vi "STS_Connect.vi"(8 "error in":errorcluster, 11 "Address Cluster out输入":T1 {"tsl_communcation_method" items=["GPIB", "C232C", "TCPIP", "USB"]; "MPM_communcation_method" items=["GPIB", "C232C", "TCPIP", "USB"]}) -> (0 "error out":errorcluster, 3 "Address Cluster out":T1 {"tsl_communcation_method" items=["GPIB", "C232C", "TCPIP", "USB"]; "MPM_communcation_method" items=["GPIB", "C232C", "TCPIP", "USB"]})   [LabVIEW 2017]
uses:
  CTL/Address Cluster.ctl
  D:/test/ILSTS/LV_IL_Sample/DLL/InstrumentDLL.dll
  DLL/InstrumentDLL.dll
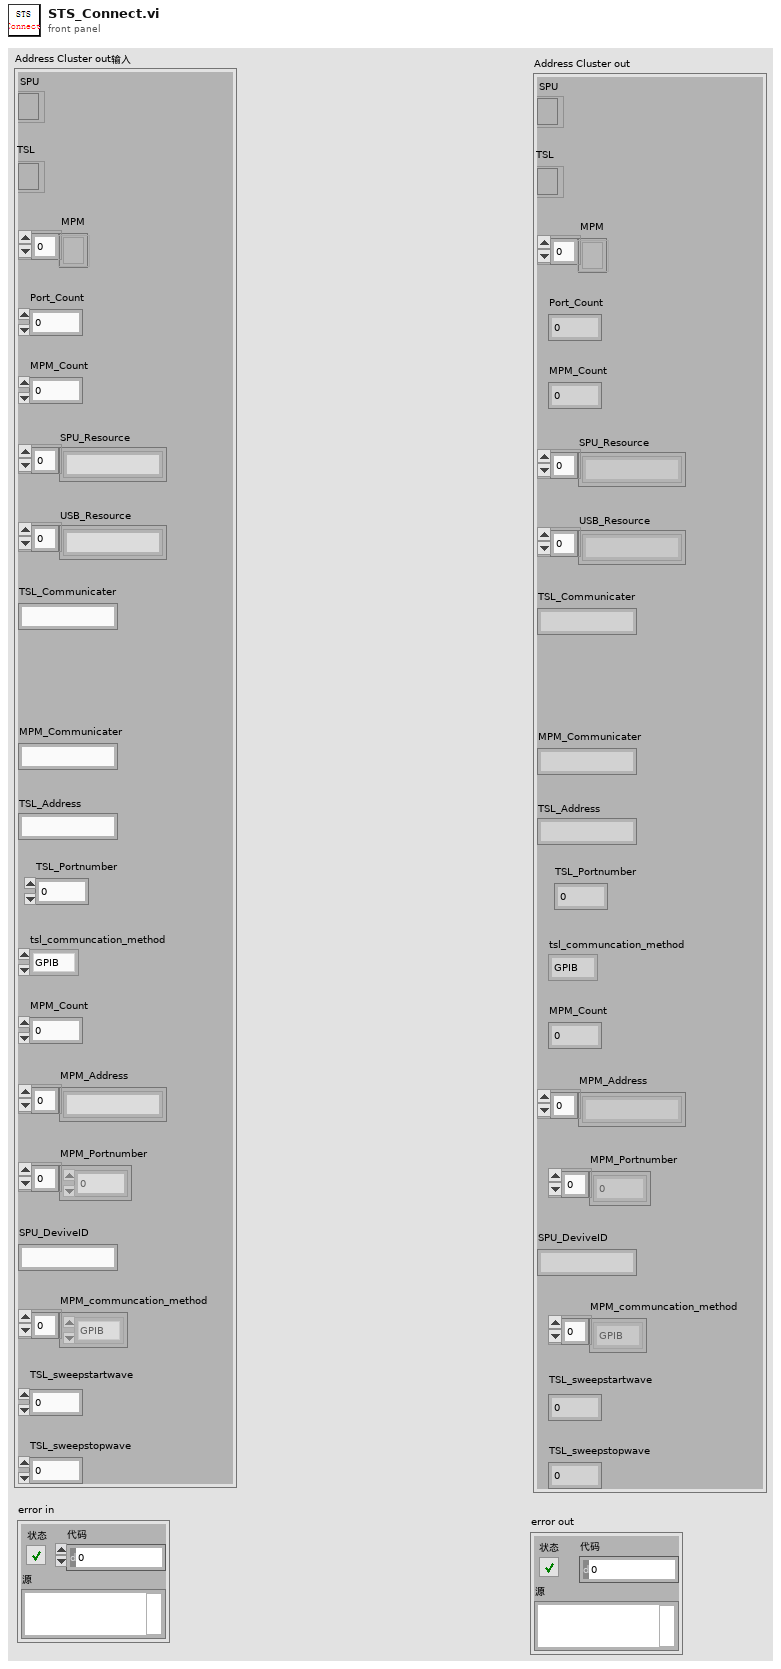
[diagram p1: front panel]
types:
  T1 = typedef "Address Cluster.ctl" = cluster{"SPU":refnum<k24>, "MPM":refnum<k24>[], "Port_Count":dbl, "MPM_Count":dbl, "SPU_Resource":string[], "USB_Resource":string[], "MPM_Communicater":string, "MPM_Count":dbl, "MPM_Address":string[], "MPM_Portnumber":dbl[], "SPU_DeviveID":string, "MPM_communcation_method":i32[], "TSL_sweepstartwave":dbl, "TSL_sweepstopwave":dbl, "TSL_Address":string, "TSL_Communicater":string, "TSL":refnum<k24>, "tsl_communcation_method":i32, "TSL_Portnumber":dbl}
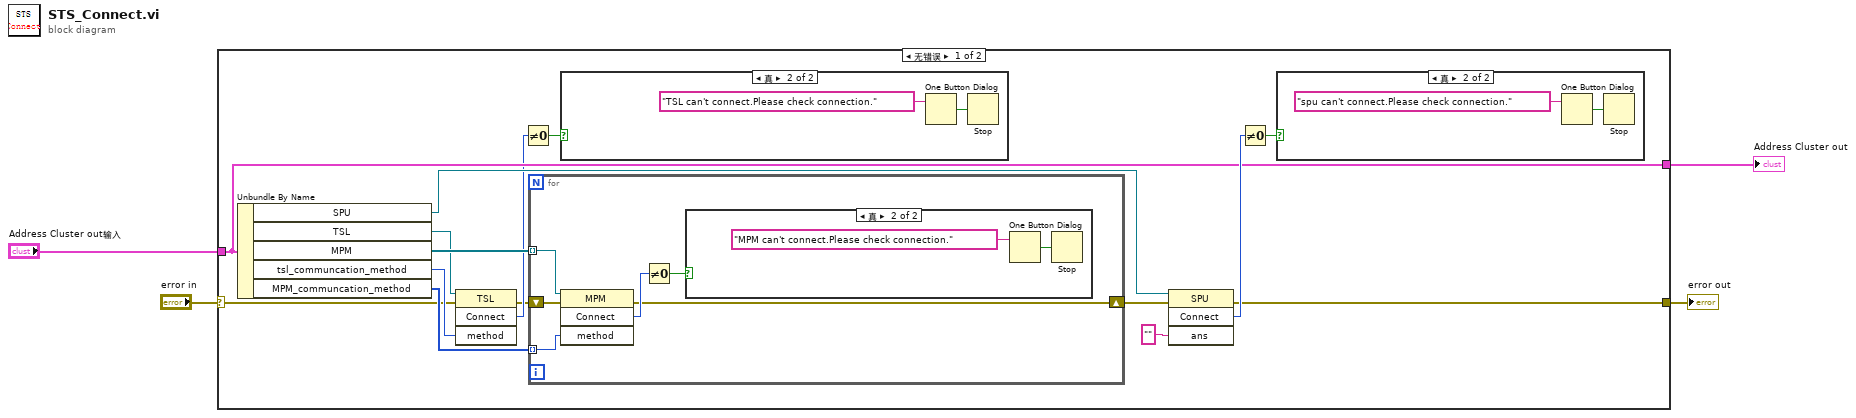
[diagram p0: block diagram]
diagram:
  n1 = case shown="无错误" "error in" {
    selector: "error in" -> [w11 w33]
    tunnel: "Address Cluster out输入" -> [w10 w32]
    tunnel: [w5 w33] -> w2
    tunnel: [w10 w32] -> w1
    frame No Error {
      n2 = Unbundle By Name(w10) -> ("SPU"=w17:refnum<k24>, "TSL"=w13:refnum<k24>, "MPM"=w15:refnum<k24>[], "tsl_communcation_method"=w14:i32, "MPM_communcation_method"=w16:i32[])
      n3 = invoke on="调用节点" class="TSL" method="Connect"(reference=w13, error in=w11, "method"=w14) -> (error out=w7:errorcluster, "Connect"=w9:i32)  [unwired: 1 in, 2 out]
      n4 = Not Equal To 0?(x=w9) -> (x != 0?=w8:bool)
      n5 = for {
        tunnel: w15 -> [w29] mode=indexing
        tunnel: w16 -> [w28] mode=indexing
        shift-right: [w25] -> w6
        shift-left: w7 -> [w24]
        n6 = invoke on="调用节点" class="MPM" method="Connect"(reference=w29, error in=w24, "method"=w28) -> (error out=w25:errorcluster, "Connect"=w26:i32)  [unwired: 1 in, 2 out]
        n7 = Not Equal To 0?(x=w26) -> (x != 0?=w27:bool)
        n8 = case shown="真" w27 {
          frame False {
          }
          frame True {
            n9 = One Button Dialog(message="MPM can't connect.Please check connection." ("消息")) -> (true=w30:bool)  [unwired: 1 in]
            n10 = Stop(stop? (T)=w30) -> ()
          }
        }
      }
      n11 = case shown="真" w8 {
        frame False {
        }
        frame True {
          n12 = One Button Dialog(message="TSL can't connect.Please check connection." ("消息")) -> (true=w20:bool)  [unwired: 1 in]
          n13 = Stop(stop? (T)=w20) -> ()
        }
      }
      n14 = invoke class="SPU" method="Connect"(reference=w17, error in=w6, "ans"="") -> (error out=w5:errorcluster, "Connect"=w19:i32)  [unwired: 1 in, 2 out]
      n15 = Not Equal To 0?(x=w19) -> (x != 0?=w18:bool)
      n16 = case shown="真" w18 {
        frame False {
        }
        frame True {
          n17 = One Button Dialog(message="spu can't connect.Please check connection." ("消息")) -> (true=w22:bool)  [unwired: 1 in]
          n18 = Stop(stop? (T)=w22) -> ()
        }
      }
    }
    frame Error {
    }
  }
  "Address Cluster out" <- w1
  "error out" <- w2
